vi "MPExxx_set_outp.vi"(2 "error in (no error)":errorcluster, 3 "Output Control":bool, 4 "VISA session":refnum<visa-resource-name>) -> (0 "error out":errorcluster, 1 "dup VISA session":refnum<visa-resource-name>)   [LabVIEW 2015]
doc: "This VI form energizes or de-energizes the power supply."
panel:
  # "MAGNA-POWER"
  # "Electronics"
  # "On"
  # "Off"
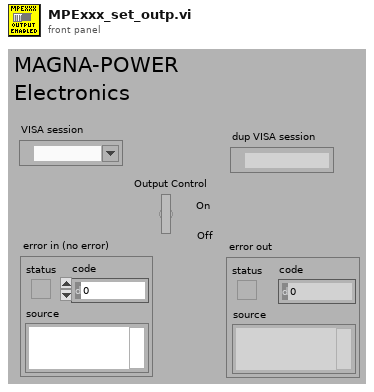
[diagram p1: front panel]
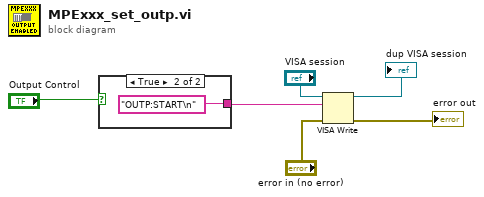
[diagram p0: block diagram]
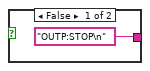
[diagram p2: hidden frame]
diagram:
  n1 = case shown="True" "Output Control" {
    tunnel: ["OUTP:STOP\n" "OUTP:START\n"] -> w5
    frame False {
    }
    frame True {
    }
  }
  n2 = VISA Write(VISA resource name="VISA session", write buffer=w5, error in (no error)="error in (no error)") -> (VISA resource name out=→"dup VISA session":refnum<visa-resource-name>, error out=→"error out":errorcluster)  [unwired: 1 out]
